vi "Aquisicao_Encoder_Simulada.vi"() -> ()   [LabVIEW 2018]
uses:
  <vilib>/ptbypt/NI_PtbyPt.lvlib
panel:
  in  "stop":bool
  out "Posição atual (°)":dbl format="%.2f"
  out "Posição Angular - Seleção de amostras mais recentes":dbl[](graph)
  out "Posição Angular":waveform(dbl)(graph)
  in  "Taxa de aquisição (Hz)":dbl
  in  "Velocidade média (°/s)":dbl(slide) scale=-100.0..100.0
  # "PROGRAMA PARA AQUISI敲O DE DADOS DO ENCODER (SIMULADO)"
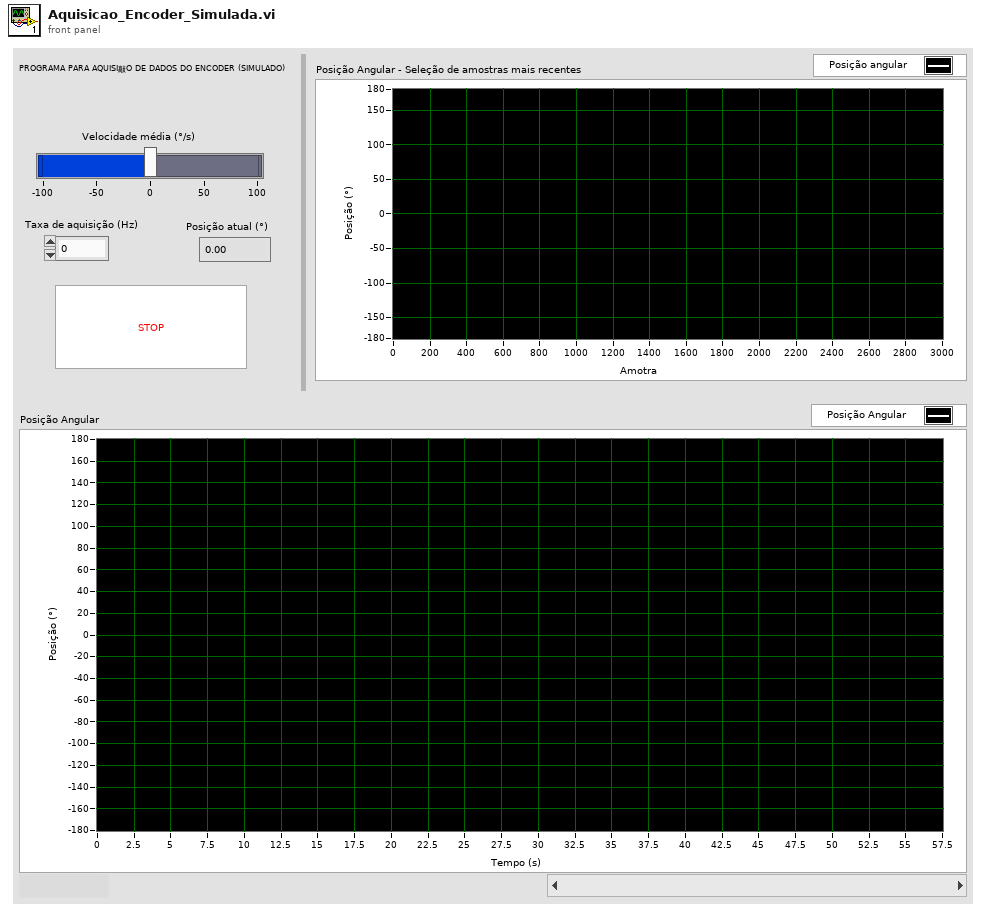
[diagram p1: front panel]
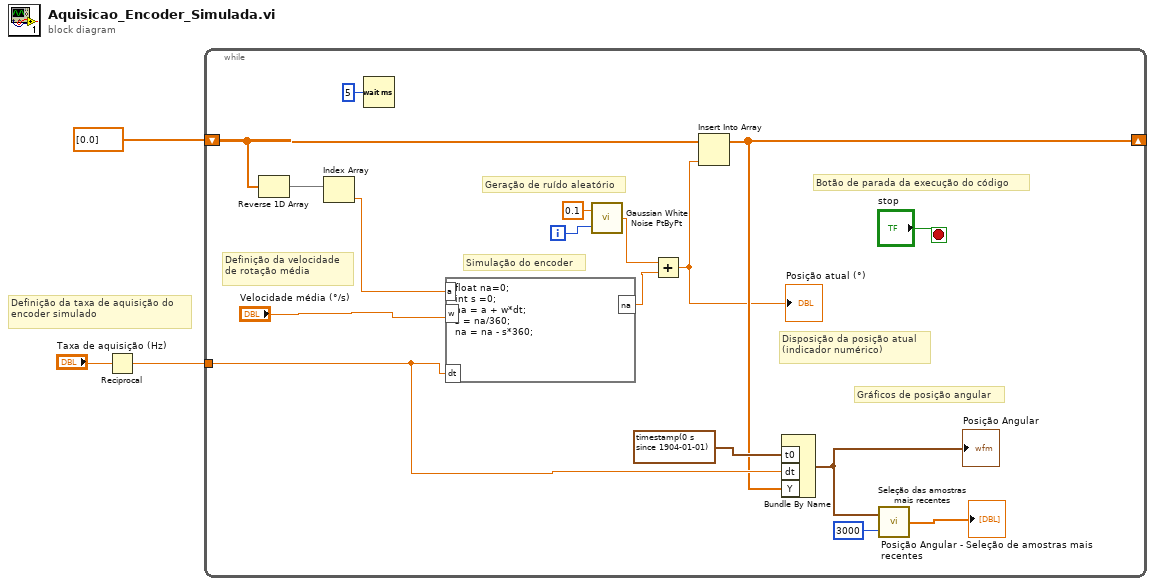
[diagram p0: block diagram]
diagram:
  # "Definição da taxa de aquisição do encoder simulado"
  n1 = Reciprocal(x="Taxa de aquisição (Hz)") -> (1/x=w1:dbl)
  n2 = while {
    tunnel: w1 -> [w12]
    shift-right: [w11] -> _
    shift-left: dbl[] [0.0] -> [w17]
    i -> [w18]
    stop <- "stop" stop-if-true
    # "Disposição da posição atual (indicador numérico)"
    # "Geração de ruído aleatório"
    # "Botão de parada da execução do código"
    # "Gráficos de posição angular"
    # "Simulação do encoder"
    # "Definição da velocidade de rotação média"
    n3 = Reverse 1D Array(array=w17) -> (reversed array=w16:dbl[])
    n4 = Index Array(array=w16) -> (element=w15:dbl)  [unwired: 1 in]
    n5 = Wait (ms)(milliseconds to wait=u32 5) -> ()  [unwired: 1 out]
    n6 = formula code="float na=0;\nint s =0;\nna = a + w*dt;\ns = na/360;\nna = na - s*360;"("a"=w15, "w"="Velocidade média (°/s)", "dt"=w12) -> ("na"=w5:dbl)
    n7 = call <vilib>:"Gaussian White Noise PtByPt.vi"("seed"=w18, "standard deviation"=0.1) -> ("Gaussian white noise"=w6:dbl)  [unwired: 1 in]
    n8 = Add(x=w6, y=w5) -> (x+y=w4:dbl)
    "Posição atual (°)" <- w4
    n9 = Insert Into Array(array=w17, new element=w4) -> (w11:dbl[])  [unwired: 1 in]
    n10 = Bundle By Name("t0"=timestamp(0 s since 1904-01-01), "dt"=w12, "Y"=w11) -> (w10:waveform(dbl))  [unwired: 1 in]
    "Posição Angular" <- w10
    n11 = call "Seleção das amostras mais recentes.vi"("Número de amostras no gráfico"=3000, "Vetor de entrada"=w10) -> ("Amostras do gráfico"=→"Posição Angular - Seleção de amostras mais recentes":dbl[])
  }
